vi "Stimulus-Create (full).vi"(6 "Rep Num":i32, 8 "error in (no error)":errorcluster, 9 "Npts":i32, 10 "Sampling Rate (Hz)":dbl, 11 "Stimulus Channel":T25(xcontrol)) -> (0 "error out":errorcluster, 1 "Sampling Rate (out)":dbl, 2 "Waveform":dbl[](graph), 3 "Stimulus Channel out":T25(xcontrol))   [LabVIEW 2020]
uses:
  Controls/Stimulus Channel (Full)/Stimulus Channel (Full).xctl
  Controls/Waveform XCtl/Waveform Enum.ctl
  Controls/Level XCtl/Level Units.ctl
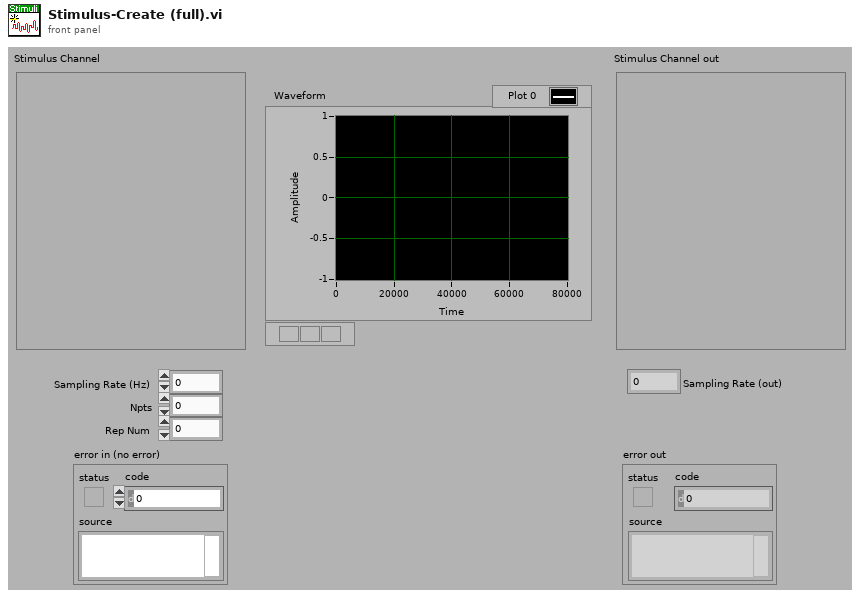
[diagram p1: front panel]
types:
  T1 = typedef "Waveform XCtl.xctl/Waveform Data.ctl" = cluster{"Type":T2, "Tone":T3, "Pulse Train":T4, "Noise":T7, "File":T8, "FMSweep":T9, "Chirp Train":T10, "Complex Tone":cluster{"Params":T12, "Data":T14}, "Moving Ripple":T15}
  T2 = typedef "Waveform Enum.ctl" = enum16{"OFF", "Tone", "Noise", "Pulse Train", "File", "FM Sweep", "Chirp Train", "Complex Tone", "FM Tone", "Moving Ripple"}
  T3 = typedef "Tone Params.ctl" = cluster{"Frequency (kHz)":dbl, "Last Freq":dbl, "Last Phase":dbl}
  T4 = typedef "Pulse Train Params.ctl" = cluster{"Pulse width (us)":dbl, "Pulse rate (Hz)":dbl, "Gap (ms)":dbl, "Polarity":T5, "PT State":T6, "Asynch":bool}
  T5 = typedef "Pulse Polarity.ctl" = enum16{"POS", "NEG", "POS-NEG", "NEG-POS"}
  T6 = typedef "PT-Continuous State.ctl" = cluster{"Template":dbl[], "Nperiod":i32, "Index":i32, "Pulse Rate (Hz)":dbl, "Phase (cycles)":dbl, "Noff":i32}
  T7 = typedef "Noise Params.ctl" = cluster{"InvFilt":bool, "Noise":dbl[], "CurPt":i32, "Aweight":bool, "Seed":i32, "afile":path}
  T8 = typedef "StimFile-Params.ctl" = cluster{"Filename":path, "Signal":dbl[], "Channel":i32, "stream":bool, "offset":i32, "nreps":i32, "loops":i32, "Randomize":bool, "order":i32[], "Seed":i32, "Tokens":i32}
  T9 = typedef "FM Sweep Params.ctl" = cluster{"Rate (oct/s)":dbl, "Fmin (Hz)":dbl, "Fmax (Hz)":dbl, "Ramp (ms)":dbl, "Linear":bool}
  T10 = typedef "Chirp Train.ctl" = cluster{"Params":T11, "Data":cluster{"WF":dbl[]}}
  T11 = typedef "Chirp Train Params.ctl" = cluster{"Fmin (kHz)":dbl, "Fmax (kHz)":dbl, "Compensate":bool, "Duration (ms)":dbl}
  T12 = typedef "CT-Params.ctl" = cluster{"F0 (Hz)":dbl, "Band":cluster{"Flow (Hz)":dbl, "Fhigh (Hz)":dbl}, "Phase":T13, "Min F0 (Hz)":dbl, "Max F0 (Hz)":dbl, "ContinRandPhase":bool, "Max peak factor":dbl, "Max mod depth":dbl, "MinHarmNum":i32, "MaxHarmNum":i32, "Level Mode":enum16{"per component", "overall rms"}, "% jitter":dbl}
  T13 = typedef "CT-Phase Enum.ctl" = enum16{"Cosine", "Random", "Alternating"}
  T14 = typedef "CT-Runtime Data.ctl" = cluster{"Ncomp":i32, "MinHarm":i32, "Phase":dbl[], "Amplitude":dbl[], "Npts/frame":i32, "Last F0":dbl, "Fmin":dbl, "Fmax":dbl, "Lslope":dbl, "randphase":bool, "overall rms":bool, "fmult":dbl[], "jittered":bool}
  T15 = typedef "Moving Ripple.ctl" = cluster{"Params":T16, "Data":T17}
  T16 = typedef "Moving Ripple.Params.ctl" = cluster{"Fmin":dbl, "Fmax":dbl, "Density":dbl, "Velocity":dbl, "Depth":dbl, "Phase":dbl, "Comp/oct":i32}
  T17 = typedef "Moving Ripple.Data.ctl" = cluster{"Freq":dbl[], "A":dbl[], "phase":dbl[], "Phase":dbl}
  T18 = typedef "Advanced Filter XCtl.xctl/Filter Data.ctl" = cluster{"Type":enum16{"Lowpass", "Highpass", "Bandpass", "Bandstop", "OFF"}, "CF (kHz)":dbl, "BW (kHz)":dbl, "Cascade":bool, "Quadrature":bool, "Scale Factor":dbl, "Stages":cluster{"IIR Filter":cluster{"filter structure":enum32{"IIR 2nd Order", "IIR 4th Order"}, "Reverse Coefficients":dbl[], "Forward Coefficients":dbl[]}, "State":dbl[]}[], "Class":enum16{"Elliptic", "Butterworth"}, "Order":i32, "BWUnits":T19}
  T19 = typedef "Filter-Bandwidth Units.ctl" = enum16{"Linear", "Octaves", "Min-Max"}
  T20 = typedef "Burst Control.xctl/Burst Data.ctl" = cluster{"Active":bool, "Delay (ms)":dbl, "Duration (ms)":dbl, "Ramp (ms)":dbl, "Rate (Hz)":dbl, "Trepeat (ms)":dbl, "Repeat":bool}
  T21 = typedef "Level XCtl.xctl/Level Data.ctl" = cluster{"Level":dbl, "Units":T22, "Max":dbl, "Multiplier":dbl, "Cal File":path, "Cal":cluster{"Freq (Hz)":dbl[], "Mag (dB SPL)":dbl[], "Phase (deg)":dbl[]}}
  T22 = typedef "Level Units.ctl" = enum16{"dB atten", "dB SPL", "dB re 1 Vrms", "dB V/Hz½", "mW", "dB HL", "Volts", "dB mW"}
  T23 = typedef "Advanced Stimulus Options.xctl/Advanced Stimulus Options.ctl" = cluster{"Rep Mask":string, "AltPol":bool, "Var":string, "Expr":string, "Persist":bool}
  T24 = typedef "SAM Params.ctl" = cluster{"Active":bool, "Frequency (Hz)":dbl, "Depth":dbl, "Init Phase (cycles)":dbl, "phase (degrees)":dbl, "Asynch":bool}
  T25 = cluster{"Waveform":T1, "Filter":T18, "Burst":T20, "Level":T21, "Name":string, "Advanced":T23, "SAM":T24}
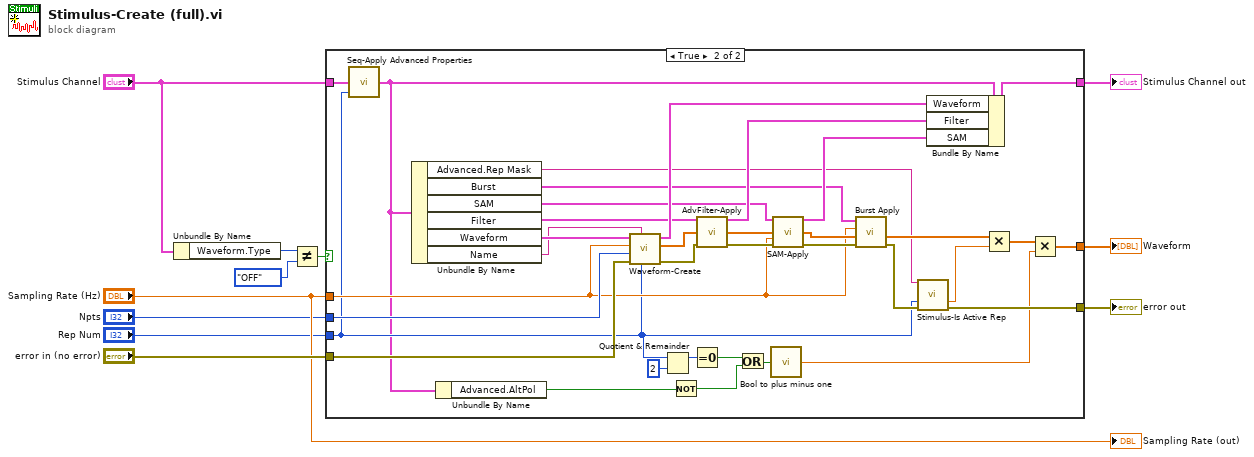
[diagram p0: block diagram]
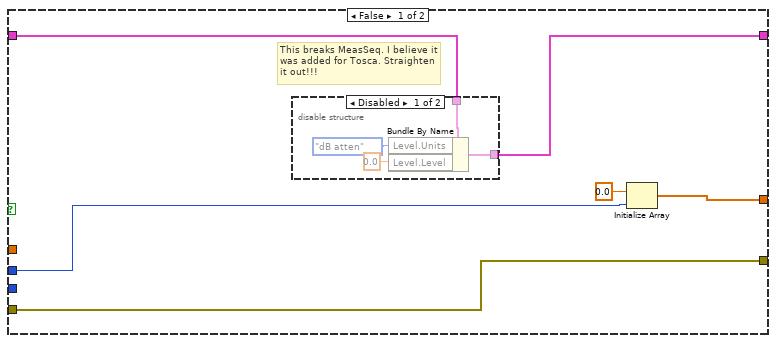
[diagram p2: hidden frame]
diagram:
  n1 = Unbundle By Name("Stimulus Channel") -> ("Waveform.Type"=w1:T2)
  n2 = Not Equal?(x=w1, y=Waveform_Enum."OFF") -> (x != y?=w5:bool)
  n3 = case shown="True" w5 {
    tunnel: "error in (no error)" -> [w17 w57]
    tunnel: "Sampling Rate (Hz)" -> [_ w41]
    tunnel: [w17 w47] -> w10
    tunnel: "Npts" -> [w15 w56]
    tunnel: [w13 w34] -> w3
    tunnel: "Stimulus Channel" -> [w16 w24]
    tunnel: [w12 w51] -> w7
    tunnel: "Rep Num" -> [_ w26]
    frame False {
      # "This breaks MeasSeq. I believe it was added for Tosca. Straighten it out!!!"
      n4 = disable-structure shown="Disabled" {
        disable-tunnel: w16 -> [w21 w22]
        disable-tunnel: [w20 w22] -> w12
        frame Disabled {
          n5 = Bundle By Name(cluster=w21, "Level.Units"=Level_Units."dB atten" ("Level.Mode"), "Level.Level"=0.0) -> (w20:T25)
        }
        frame Enabled {
        }
      }
      n6 = Initialize Array(0.0 ("element"), w15) -> (w13:dbl[])
    }
    frame True {
      n7 = call "Seq-Apply Advanced Properties.vi"("Rep"=w26, "Stimulus Channel in"=w24) -> ("Stimulus Channel out"=w25:T25)  [unwired: 3 in]
      n8 = Unbundle By Name(w25) -> ("Advanced.Rep Mask"=w32:string, "Burst"=w31:T20, "SAM"=w30:T24, "Filter"=w29:T18, "Waveform"=w28:T1, "Name"=w23:string)
      n9 = Unbundle By Name(w25) -> ("Advanced.AltPol"=w27:bool)
      n10 = call "Waveform-Create.vi"("Rep Num"=w26, "Name"=w23, "error in (no error)"=w57, "Npts"=w56, "Sampling Rate (Hz)"=w41, "Waveform"=w28) -> ("error out"=w53:errorcluster, "Signal"=w54:dbl[], "Waveform out"=w50:T1)  [unwired: 3 in]
      n11 = Quotient & Remainder(x=w26, y=2) -> (x-y*floor(x/y)=w38:i32)  [unwired: 1 out]
      n12 = Not(x=w27) -> (.not. x?=w36:bool)
      n13 = Equal To 0?(x=w38) -> (x = 0?=w37:bool)
      n14 = call "AdvFilter-Apply.vi"("Filter"=w29, "X"=w54, "error in (no error)"=w53) -> ("Filter out"=w52:T18, "Filtered X"=w43:dbl[], "error out"=w44:errorcluster)  [unwired: 10 in]
      n15 = Or(x=w37, y=w36) -> (x .or. y?=w35:bool)
      n16 = call "Bool to plus minus one.vi"("Boolean"=w35) -> ("Numeric"=w33:dbl)
      n17 = call "SAM-Apply.vi"("SAM In"=w30, "X"=w43, "Sampling Rate (Hz)"=w41, "error in (no error)"=w44) -> ("SAM Out"=w40:T24, "Modulated X"=w42:dbl[], "error out"=w45:errorcluster)  [unwired: 9 in]
      n18 = call "Burst Apply.vi"("error in (no error)"=w45, "Waveform in"=w42, "Sampling Rate (Hz)"=w41, "Burst"=w31) -> ("error out"=w48:errorcluster, "Gated waveform"=w55:dbl[])  [unwired: 6 in]
      n19 = call "Stimulus-Is Active Rep.vi"("Advanced.Rep Mask"=w32, "Rep Num"=w26, "error in (no error)"=w48) -> ("Multiplier"=w46:dbl, "error out"=w47:errorcluster)  [unwired: 10 in, 1 out]
      n20 = Bundle By Name(cluster=w25, "Waveform"=w50, "Filter"=w52, "SAM"=w40) -> (w51:T25)
      n21 = Multiply(x=w55, y=w46) -> (x*y=w49:dbl[])
      n22 = Multiply(x=w49, y=w33) -> (x*y=w34:dbl[])
    }
  }
  "error out" <- w10
  "Waveform" <- w3
  "Stimulus Channel out" <- w7
  "Sampling Rate (out)" <- "Sampling Rate (Hz)"
